vi "Initialize.vi"(8 "error in (no error)":errorcluster, 11 "Masterv2 in":refnum<class "Masterv2.lvclass">) -> (0 "error out":errorcluster, 3 "Masterv2 out":refnum<class "Masterv2.lvclass">)   [LabVIEW 2014, in "Main Libraryv2.lvlib" / "Masterv2.lvclass"]
uses:
  Master/Masterv2.lvclass
  Stryker/Drying Machine 06.20.2015/CONTROL/statedef.ctl
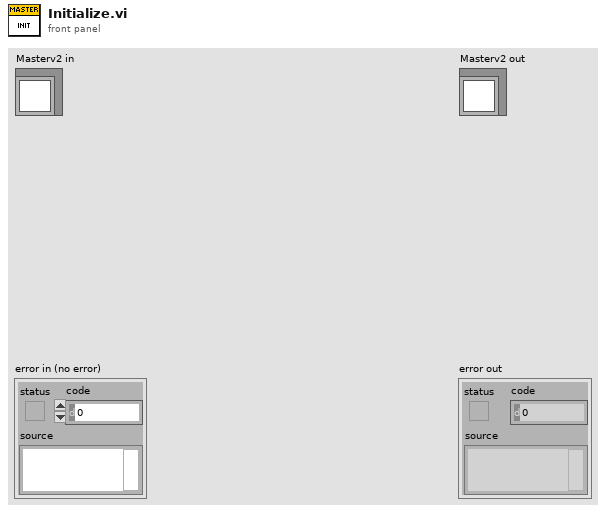
[diagram p1: front panel]
types:
  T1 = typedef "Files Library.lvlib/CONTROL LIBRARY.lvlib/statedef.ctl" = cluster{"State":string, "Data":variant}
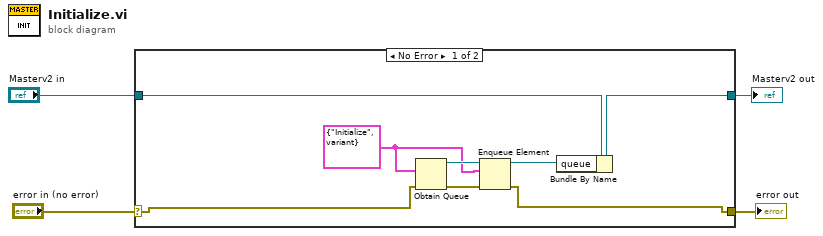
[diagram p0: block diagram]
diagram:
  n1 = case shown="No Error" "error in (no error)" {
    selector: "error in (no error)" -> [w7 w14]
    tunnel: [w8 w14] -> w3
    tunnel: [w5 w13] -> w1
    tunnel: "Masterv2 in" -> [w6 w13]
    frame No Error {
      w10 = T1 {"State"="Initialize", "Data"=variant} ("StateDatas")
      n2 = Obtain Queue(element data type=w10, error in (no error)=w7) -> (queue out=w12:refnum<queue>, error out=w9:errorcluster)  [unwired: 3 in, 1 out]
      n3 = Enqueue Element(queue=w12, element=w10, error in (no error)=w9) -> (queue out=w11:refnum<queue>, error out=w8:errorcluster)  [unwired: 1 in, 1 out]
      n4 = Bundle By Name(cluster=w6, "queue"=w11) -> (w5:refnum<class "Masterv2.lvclass">)
    }
    frame Error {
    }
  }
  "error out" <- w3
  "Masterv2 out" <- w1
